vi "_API_BINANCE_POST_USDT_FUTURES_NewOrder.vi"(0 "BinanceAPI in":refnum<class "BinanceAPI_.lvclass">, 5 "NewOrder":T1={"symbol"="NaN", "side"=enum."NaN", "type"=enum."NaN", "timeInForce"=enum."NaN", "quantity"=nan, "price"=nan, "newClientOrderId"="NaN", "stopPrice"=nan, "positionSide"=enum."NaN", "reduceOnly"="NaN", "closePosition"="NaN", "activationPrice"=0.0, "callbackRate"=0, "workingType"=enum."NaN", "priceProtect"="NaN", "newOrderRespType"=enum."NaN", "recvWindow"=5000}, 11 "error in (no error)":errorcluster) -> (4 "BinanceAPI out":refnum<class "BinanceAPI_.lvclass">, 14 "Body":string, 15 "error IO":errorcluster)   [LabVIEW 2022 SP3, in "BinanceAPI_.lvclass"]
doc: "https://binance-docs.github.io/apidocs/futures/en/#new-order-trade"
uses:
  BinanceAPI_.lvclass
  BinanceAPI_.lvclass/BinanceAPI_.ctl
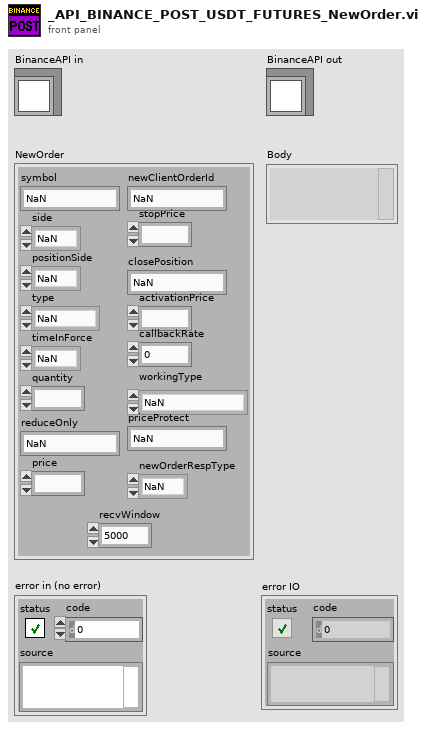
[diagram p1: front panel]
types:
  T1 = cluster{"symbol":string, "side":enum16{"NaN", "SELL", "BUY"}, "type":enum16{"NaN", "LIMIT", "MARKET", "STOP", "STOP_MARKET", "TAKE_PROFIT", "TAKE_PROFIT_MARKET", "TRAILING_STOP_MARKET"}, "timeInForce":enum16{"NaN", "GTC", "IOC", "FOK"}, "quantity":ext, "price":ext, "newClientOrderId":string, "stopPrice":ext, "positionSide":enum16{"NaN", "BOTH", "LONG", "SHORT"}, "reduceOnly":string, "closePosition":string, "activationPrice":ext, "callbackRate":i32, "workingType":enum16{"NaN", "MARK_PRICE", "CONTRACT_PRICE"}, "priceProtect":string, "newOrderRespType":enum16{"NaN", "ACK", "RESULT", "FULL"}, "recvWindow":i32}
  T2 = enum16{"SPOT", "USDT_FUTURES", "COIN_FUTURES", "VANILLA"}
  T3 = enum16{"NaN", "LIMIT", "MARKET", "STOP", "STOP_MARKET", "TAKE_PROFIT", "TAKE_PROFIT_MARKET", "TRAILING_STOP_MARKET"}
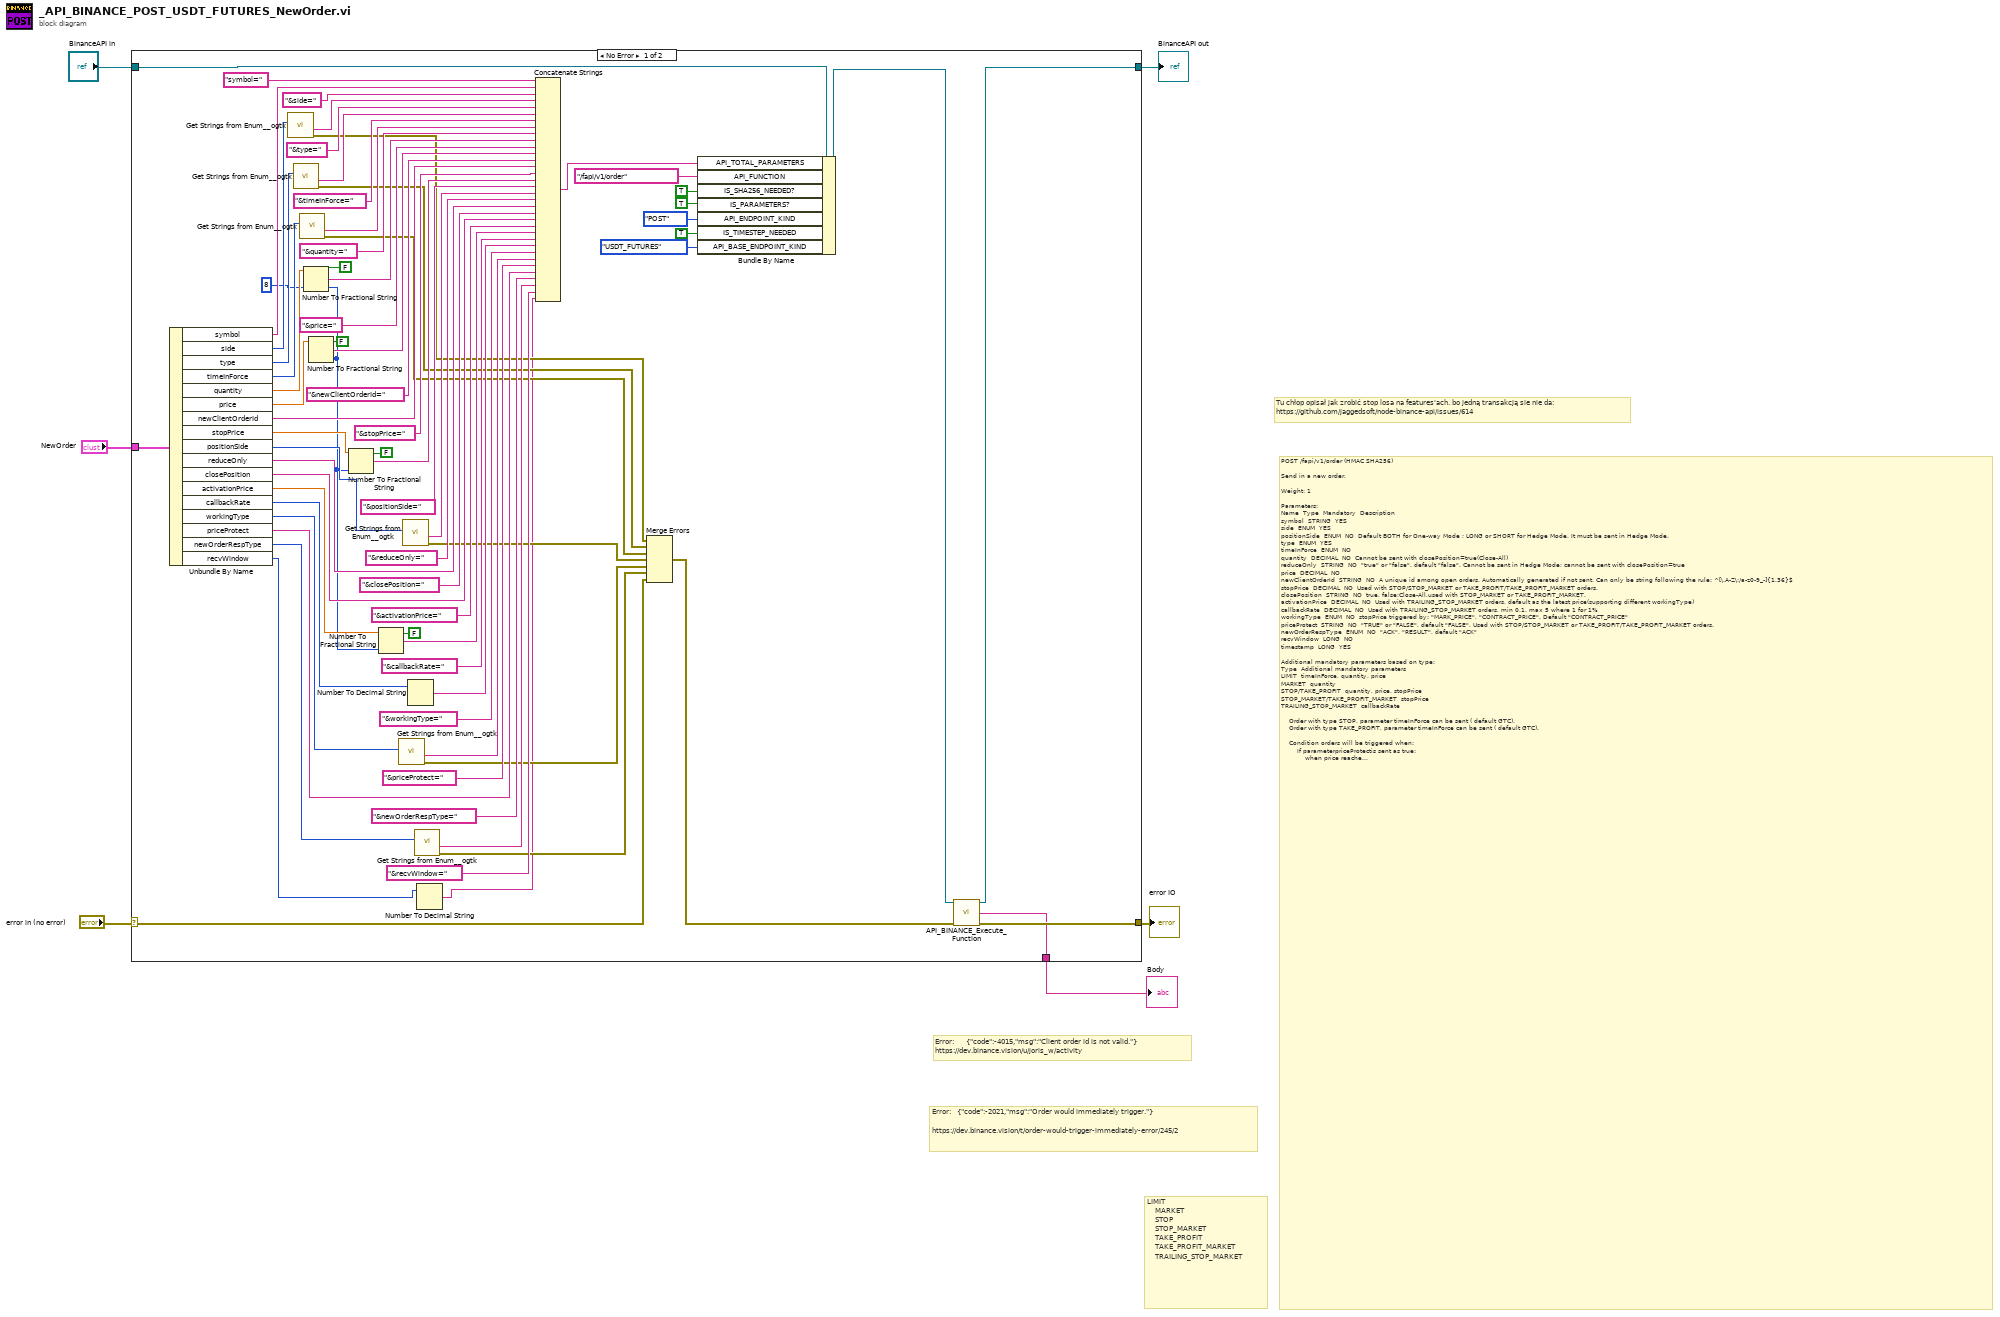
[diagram p0: block diagram]
diagram:
  # "Error:      {\"code\":-4015,\"msg\":\"Client order id is not valid.\"}\nhttps://dev.binance.vision/u/joris_w/activity"
  # "Error:   {\"code\":-2021,\"msg\":\"Order would immediately trigger.\"}\n\nhttps://dev.binance.vision/t/order-would-trigger-immediately-error/245/2"
  # "LIMIT\n    MARKET\n    STOP\n    STOP_MARKET\n    TAKE_PROFIT\n    TAKE_PROFIT_MARKET\n    TRAILING_STOP_MARKET"
  # "Tu chłop opisał jak zrobić stop losa na features'ach. bo jedną transakcją sie nie da:\nhttps://github.com/jaggedsoft/node-binance-api/issues/614"
  # "POST /fapi/v1/order (HMAC SHA256)\n\nSend in a new order.\n\nWeight: 1\n\nParameters:\nName \tType \tMandatory \tDescription\nsymbol \tSTRING \tYES \t\nside \tENUM \tYES \t\npositionSide \tENUM \tNO \tDefault BOTH for One-way Mode ; LONG or SHORT for Hedge Mode. It must be sent in Hedge Mode.\ntype \tENUM \tYES \t\ntimeInForce \tENUM \tNO \t\nquantity \tDECIMAL \tNO \tCannot be sent with closePosition=true(Close-All)\nreduceOnly \tSTRING \tNO \t\"true\" or \"false\". default \"false\". Cannot be sent in Hedge Mode; cannot be sent with closePosition=true\nprice \tDECIMAL \tNO \t\nnewClientOrderId \tSTRING \tNO \tA unique id among open orders. Automatically generated if not sent. Can only be string following the rule: ^[\\.A-Z\\:/a-z0-9_-]{1,36}$\nstopPrice \tDECIMAL \tNO \tUsed with STOP/STOP_MARKET or TAKE_PROFIT/TAKE_PROFIT_MARKET orders.\nclosePosition \tSTRING \tNO \ttrue, false;Close-All,used with STOP_MARKET or TAKE_PROFIT_MARKET.\nactivationPrice \tDECIMAL \tNO \tUsed with TRAILING_STOP_MARKET orders, default as the latest price(supporting different workingType)\ncallbackRate \tDECIMAL \tNO \tUsed with TRAILING_STOP_MARKET orders, min 0.1, max 5 where 1 for 1%\nworkingType \tENUM \tNO \tstopPrice triggered by: \"MARK_PRICE\", \"CONTRACT_PRICE\". Default \"CONTRACT_PRICE\"\npriceProtect \tSTRING \tNO \t\"TRUE\" or \"FALSE\", default \"FALSE\". Used with STOP/STOP_MARKET or TAKE_PROFIT/TAKE_PROFIT_MARKET orders.\nnewOrderRespType \tENUM \tNO \t\"ACK\", \"RESULT\", default \"ACK\"\nrecvWindow \tLONG \tNO \t\ntimestamp \tLONG \tYES \t\n\nAdditional mandatory parameters based on type:\nType \tAdditional mandatory parameters\nLIMIT \ttimeInForce, quantity, price\nMARKET \tquantity\nSTOP/TAKE_PROFIT \tquantity, price, stopPrice\nSTOP_MARKET/TAKE_PROFIT_MARKET \tstopPrice\nTRAILING_STOP_MARKET \tcallbackRate\n\n    Order with type STOP, parameter timeInForce can be sent ( default GTC).\n    Order with type TAKE_PROFIT, parameter timeInForce can be sent ( default GTC).\n\n    Condition orders will be triggered when:\n        If parameterpriceProtectis sent as true:\n            when price reaches the stopPrice ,the difference rate between \"MARK_PRICE\" and \"CONTRACT_PRICE\" cannot be larger than the \"triggerProtect\" of the symbol\n            \"triggerProtect\" of a symbol can be got from GET /fapi/v1/exchangeInfo\n        STOP, STOP_MARKET:\n            BUY: latest price (\"MARK_PRICE\" or \"CONTRACT_PRICE\") >= stopPrice\n            SELL: latest price (\"MARK_PRICE\" or \"CONTRACT_PRICE\") <= stopPrice\n        TAKE_PROFIT, TAKE_PROFIT_MARKET:\n            BUY: latest price (\"MARK_PRICE\" or \"CONTRACT_PRICE\") <= stopPrice\n            SELL: latest price (\"MARK_PRICE\" or \"CONTRACT_PRICE\") >= stopPrice\n        TRAILING_STOP_MARKET:\n            BUY: the lowest price after order placed <= activationPrice, and the latest price >= the lowest price * (1 + callbackRate)\n            SELL: the highest price after order placed >= activationPrice, and the latest price <= the highest price * (1 - callbackRate)\n\n    For TRAILING_STOP_MARKET, if you got such error code.\n    {\"code\": -2021, \"msg\": \"Order would immediately trigger.\"}\n    means that the parameters you send do not meet the following requirements:\n        BUY: activationPrice should be smaller than latest price.\n        SELL: activationPrice should be larger than latest price.\n\n    If newOrderRespType is sent as RESULT :\n        MARKET order: the final FILLED result of the order will be return directly.\n        LIMIT order with special timeInForce: the final status result of the order(FILLED or EXPIRED) will be returned directly.\n\n    STOP_MARKET, TAKE_PROFIT_MARKET with closePosition=true:\n        Follow the same rules for condition orders.\n        If triggered,close all current long position( if SELL) or current short position( if BUY).\n        Cannot be used with quantity paremeter\n        Cannot be used with reduceOnly parameter\n        In Hedge Mode,cannot be used with BUY orders in LONG position side. and cannot be used with SELL orders in SHORT position side"
  n1 = case shown="No Error" "error in (no error)" {
    selector: "error in (no error)" -> [w71 w80]
    tunnel: [w66 w80] -> w3
    tunnel: [w68 w79] -> w1
    tunnel: "BinanceAPI in" -> [w72 w79]
    tunnel: "NewOrder" -> [w75 _]
    tunnel: [w7 _] -> w4
    frame No Error {
      w32 = i16 8 ("precision (6)")
      n2 = Unbundle By Name(w75) -> ("symbol"=w63:string, "side"=w61:enum16{"NaN", "SELL", "BUY"}, "type"=w58:T3, "timeInForce"=w54:enum16{"NaN", "GTC", "IOC", "FOK"}, "quantity"=w49:ext, "price"=w48:ext, "newClientOrderId"=w46:string, "stopPrice"=w43:ext, "positionSide"=w41:enum16{"NaN", "BOTH", "LONG", "SHORT"}, "reduceOnly"=w38:string, "closePosition"=w36:string, "activationPrice"=w33:ext, "callbackRate"=w28:i32, "workingType"=w25:enum16{"NaN", "MARK_PRICE", "CONTRACT_PRICE"}, "priceProtect"=w23:string, "newOrderRespType"=w21:enum16{"NaN", "ACK", "RESULT", "FULL"}, "recvWindow"=w9:i32)
      n3 = call <userlib>:"Get Strings from Enum__ogtk.vi"("Enum"=w61) -> ("error out"=w10:errorcluster, "String Value"=w60:string)  [unwired: 7 in, 2 out]
      n4 = call <userlib>:"Get Strings from Enum__ogtk.vi"("Enum"=w58) -> ("error out"=w11:errorcluster, "String Value"=w57:string)  [unwired: 7 in, 2 out]
      n5 = call <userlib>:"Get Strings from Enum__ogtk.vi"("Enum"=w54) -> ("error out"=w12:errorcluster, "String Value"=w55:string)  [unwired: 7 in, 2 out]
      n6 = Number To Fractional String(use system decimal point (T)=FALSE, number=w49, precision (6)=w32) -> (F-format string=w52:string)  [unwired: 1 in]
      n7 = Number To Fractional String(use system decimal point (T)=FALSE, number=w48, precision (6)=w32) -> (F-format string=w50:string)  [unwired: 1 in]
      n8 = Number To Fractional String(use system decimal point (T)=FALSE, number=w43, precision (6)=w32) -> (F-format string=w45:string)  [unwired: 1 in]
      n9 = Number To Fractional String(use system decimal point (T)=FALSE, number=w33, precision (6)=w32) -> (F-format string=w35:string)  [unwired: 1 in]
      n10 = call <userlib>:"Get Strings from Enum__ogtk.vi"("Enum"=w25) -> ("error out"=w14:errorcluster, "String Value"=w26:string)  [unwired: 7 in, 2 out]
      n11 = call <userlib>:"Get Strings from Enum__ogtk.vi"("Enum"=w41) -> ("error out"=w13:errorcluster, "String Value"=w40:string)  [unwired: 7 in, 2 out]
      n12 = Number To Decimal String(number=w28) -> (decimal integer string=w29:string)  [unwired: 1 in]
      n13 = call <userlib>:"Get Strings from Enum__ogtk.vi"("Enum"=w21) -> ("error out"=w15:errorcluster, "String Value"=w20:string)  [unwired: 7 in, 2 out]
      n14 = Number To Decimal String(number=w9) -> (decimal integer string=w8:string)  [unwired: 1 in]
      n15 = Concatenate Strings("symbol=" ("Symbol"), w63, "&side=" ("Symbol"), w60, "&type=" ("Symbol"), w57, "&timeInForce=" ("Symbol"), w55, "&quantity=" ("Symbol"), w52, "&price=" ("Symbol"), w50, "&newClientOrderId=" ("Symbol"), w46, "&stopPrice=" ("Symbol"), w45, "&positionSide=" ("Symbol"), w40, "&reduceOnly=" ("Symbol"), w38, "&closePosition=" ("Symbol"), w36, "&activationPrice=" ("Symbol"), w35, "&callbackRate=" ("Symbol"), w29, "&workingType=" ("Symbol"), w26, "&priceProtect=" ("Symbol"), w23, "&newOrderRespType=" ("Symbol"), w20, "&recvWindow=" ("Symbol"), w8) -> (w74:string)
      n16 = Merge Errors(w10, w11, w12, w13, w14, w15, w71) -> (w67:errorcluster)
      n17 = Bundle By Name(cluster=w72, "API_TOTAL_PARAMETERS"=w74, "API_FUNCTION"="/fapi/v1/order", "IS_SHA256_NEEDED?"=TRUE, "IS_PARAMETERS?"=TRUE, "API_ENDPOINT_KIND"=enum16{"POST", "DELETE", "GET", "PUT"}."POST", "IS_TIMESTEP_NEEDED"=TRUE ("IS_PARAMETERS?"), "API_BASE_ENDPOINT_KIND"=T2."USDT_FUTURES") -> (w69:refnum<class "BinanceAPI_.lvclass">)
      n18 = call "API_BINANCE_Execute_Function.vi"("BinanceAPI in"=w69, "error in (no error)"=w67) -> ("BinanceAPI out"=w68:refnum<class "BinanceAPI_.lvclass">, "Body"=w7:string, "error out"=w66:errorcluster)  [unwired: 9 in, 2 out]
    }
    frame Error {
    }
  }
  "Body" <- w4
  "error IO" <- w3
  "BinanceAPI out" <- w1
